vi "median and average.vi"(0 "sensor 1":dbl[](array[numeric]), 1 "sensor2":dbl[](array[numeric]), 2 "sensor3":dbl[](array[numeric]), 3 "sensor 4":dbl[](array[numeric]), 4 "sensor 5":dbl[](array[numeric]), 5 "sensor 6":dbl[](array[numeric]), 6 "sensor 7":dbl[](array[numeric]), 7 "sensor 8":dbl[](array[numeric]), 9 "sensor 9":dbl[](array[numeric])) -> (19 "9":dbl caption="均值9" format="%0.2f", 20 "1":dbl caption="均值1" format="%0.2f", 21 "2":dbl caption="均值2" format="%0.2f", 22 "3":dbl caption="均值3" format="%0.2f", 23 "4":dbl caption="均值4" format="%0.2f", 24 "5":dbl caption="均值5" format="%0.4f", 25 "6":dbl caption="均值6" format="%0.2f", 26 "7":dbl caption="均值7" format="%0.2f", 27 "8":dbl caption="均值8" format="%0.2f")   [LabVIEW 2017]
uses:
  <vilib>/Analysis/baseanly.llb/Mean (DBL).vi
  <vilib>/Analysis/NI_AALBase.lvlib
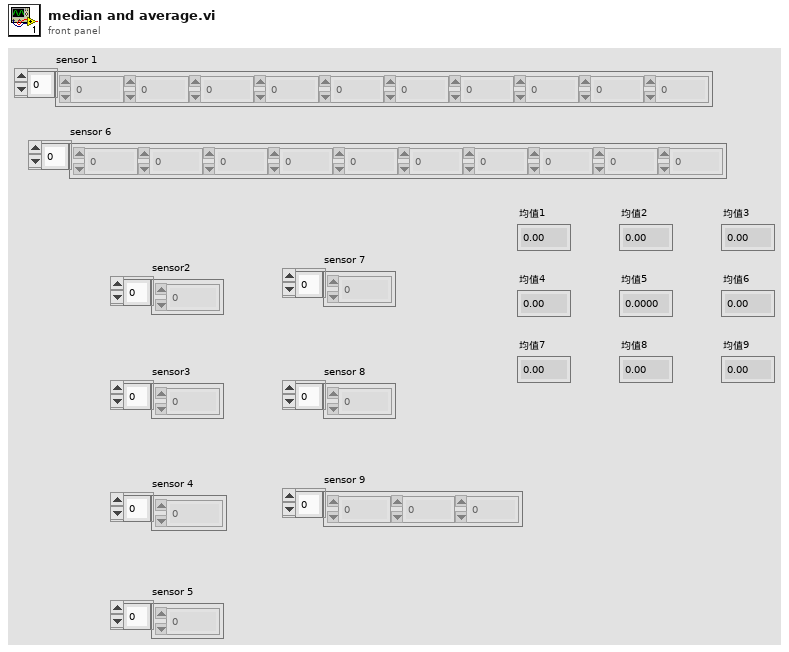
[diagram p1: front panel]
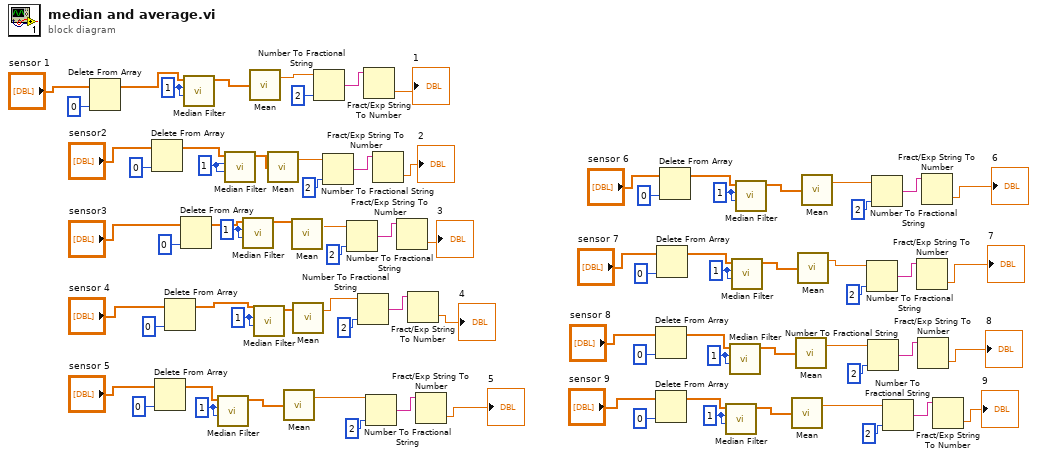
[diagram p0: block diagram]
diagram:
  w65 = 1 ("left rank")
  w66 = 1 ("left rank")
  w69 = 1 ("left rank")
  w70 = 1 ("left rank")
  w73 = 1 ("left rank")
  w74 = 1 ("left rank")
  w77 = 1 ("left rank")
  w78 = 1 ("left rank")
  w81 = 1 ("left rank")
  n1 = Delete From Array(array="sensor 1", index=0 ("索引")) -> (array with subset deleted=w61:dbl[])  [unwired: 1 in, 1 out]
  n2 = Delete From Array(array="sensor2", index=0 ("索引")) -> (array with subset deleted=w58:dbl[])  [unwired: 1 in, 1 out]
  n3 = Delete From Array(array="sensor 5", index=0 ("索引")) -> (array with subset deleted=w49:dbl[])  [unwired: 1 in, 1 out]
  n4 = Delete From Array(array="sensor 4", index=0 ("索引")) -> (array with subset deleted=w52:dbl[])  [unwired: 1 in, 1 out]
  n5 = Delete From Array(array="sensor3", index=0 ("索引")) -> (array with subset deleted=w55:dbl[])  [unwired: 1 in, 1 out]
  n6 = call <vilib>:"Median Filter.vi"("right rank"=w81, "left rank"=w81, "X"=w61) -> ("Filtered X"=w80:dbl[])  [unwired: 7 in, 1 out]
  n7 = call <vilib>:"Median Filter.vi"("right rank"=w73, "left rank"=w73, "X"=w49) -> ("Filtered X"=w72:dbl[])  [unwired: 7 in, 1 out]
  n8 = call <vilib>:"Median Filter.vi"("right rank"=w78, "left rank"=w78, "X"=w58) -> ("Filtered X"=w79:dbl[])  [unwired: 7 in, 1 out]
  n9 = call <vilib>:"Median Filter.vi"("right rank"=w77, "left rank"=w77, "X"=w55) -> ("Filtered X"=w76:dbl[])  [unwired: 7 in, 1 out]
  n10 = call-poly <vilib>:"Mean.vi"("X"=w80) -> ("mean"=w36:dbl)  [unwired: 1 out]
  n11 = call <vilib>:"Median Filter.vi"("right rank"=w74, "left rank"=w74, "X"=w52) -> ("Filtered X"=w75:dbl[])  [unwired: 7 in, 1 out]
  n12 = call-poly <vilib>:"Mean.vi"("X"=w79) -> ("mean"=w30:dbl)  [unwired: 1 out]
  n13 = call-poly <vilib>:"Mean.vi"("X"=w72) -> ("mean"=w18:dbl)  [unwired: 1 out]
  n14 = call-poly <vilib>:"Mean.vi"("X"=w76) -> ("mean"=w26:dbl)  [unwired: 1 out]
  n15 = call-poly <vilib>:"Mean.vi"("X"=w75) -> ("mean"=w22:dbl)  [unwired: 1 out]
  n16 = Number To Fractional String(number=w36, precision (6)=i16 2 ("精度(6)")) -> (F-format string=w34:string)  [unwired: 2 in]
  n17 = Number To Fractional String(number=w30, precision (6)=i16 2 ("精度(6)")) -> (F-format string=w32:string)  [unwired: 2 in]
  n18 = Number To Fractional String(number=w26, precision (6)=i16 2 ("精度(6)")) -> (F-format string=w28:string)  [unwired: 2 in]
  n19 = Number To Fractional String(number=w22, precision (6)=i16 2 ("精度(6)")) -> (F-format string=w24:string)  [unwired: 2 in]
  n20 = Fract/Exp String To Number(string=w34) -> (number=→"1":dbl)  [unwired: 3 in, 1 out]
  n21 = Number To Fractional String(number=w18, precision (6)=i16 2 ("精度(6)")) -> (F-format string=w20:string)  [unwired: 2 in]
  n22 = Fract/Exp String To Number(string=w32) -> (number=→"2":dbl)  [unwired: 3 in, 1 out]
  n23 = Fract/Exp String To Number(string=w28) -> (number=→"3":dbl)  [unwired: 3 in, 1 out]
  n24 = Fract/Exp String To Number(string=w24) -> (number=→"4":dbl)  [unwired: 3 in, 1 out]
  n25 = Fract/Exp String To Number(string=w20) -> (number=→"5":dbl)  [unwired: 3 in, 1 out]
  n26 = Delete From Array(array="sensor 8", index=0 ("索引")) -> (array with subset deleted=w40:dbl[])  [unwired: 1 in, 1 out]
  n27 = Delete From Array(array="sensor 9", index=0 ("索引")) -> (array with subset deleted=w37:dbl[])  [unwired: 1 in, 1 out]
  n28 = Delete From Array(array="sensor 7", index=0 ("索引")) -> (array with subset deleted=w43:dbl[])  [unwired: 1 in, 1 out]
  n29 = Delete From Array(array="sensor 6", index=0 ("索引")) -> (array with subset deleted=w46:dbl[])  [unwired: 1 in, 1 out]
  n30 = call <vilib>:"Median Filter.vi"("right rank"=w65, "left rank"=w65, "X"=w37) -> ("Filtered X"=w64:dbl[])  [unwired: 7 in, 1 out]
  n31 = call <vilib>:"Median Filter.vi"("right rank"=w66, "left rank"=w66, "X"=w40) -> ("Filtered X"=w67:dbl[])  [unwired: 7 in, 1 out]
  n32 = call <vilib>:"Median Filter.vi"("right rank"=w69, "left rank"=w69, "X"=w43) -> ("Filtered X"=w68:dbl[])  [unwired: 7 in, 1 out]
  n33 = call <vilib>:"Median Filter.vi"("right rank"=w70, "left rank"=w70, "X"=w46) -> ("Filtered X"=w71:dbl[])  [unwired: 7 in, 1 out]
  n34 = call-poly <vilib>:"Mean.vi"("X"=w64) -> ("mean"=w2:dbl)  [unwired: 1 out]
  n35 = call-poly <vilib>:"Mean.vi"("X"=w67) -> ("mean"=w4:dbl)  [unwired: 1 out]
  n36 = call-poly <vilib>:"Mean.vi"("X"=w68) -> ("mean"=w6:dbl)  [unwired: 1 out]
  n37 = call-poly <vilib>:"Mean.vi"("X"=w71) -> ("mean"=w8:dbl)  [unwired: 1 out]
  n38 = Number To Fractional String(number=w6, precision (6)=i16 2 ("精度(6)")) -> (F-format string=w14:string)  [unwired: 2 in]
  n39 = Number To Fractional String(number=w4, precision (6)=i16 2 ("精度(6)")) -> (F-format string=w12:string)  [unwired: 2 in]
  n40 = Number To Fractional String(number=w8, precision (6)=i16 2 ("精度(6)")) -> (F-format string=w16:string)  [unwired: 2 in]
  n41 = Number To Fractional String(number=w2, precision (6)=i16 2 ("精度(6)")) -> (F-format string=w10:string)  [unwired: 2 in]
  n42 = Fract/Exp String To Number(string=w14) -> (number=→"7":dbl)  [unwired: 3 in, 1 out]
  n43 = Fract/Exp String To Number(string=w12) -> (number=→"8":dbl)  [unwired: 3 in, 1 out]
  n44 = Fract/Exp String To Number(string=w16) -> (number=→"6":dbl)  [unwired: 3 in, 1 out]
  n45 = Fract/Exp String To Number(string=w10) -> (number=→"9":dbl)  [unwired: 3 in, 1 out]
